vi "Go to Localize.vi"(8 "error in (no error)":errorcluster, 11 "CommonState in":refnum<class "CoordinatorState.lvclass">) -> (0 "error out":errorcluster, 3 "CommonState out":refnum<class "State Actor.lvclass">)   [LabVIEW 2014, in "States.lvlib" / "CoordinatorState.lvclass"]
uses:
  CoordinatorState.lvclass
  <vilib>/NI/Actors/State Actor/State Actor/State Actor.lvclass
  Localize/Localize.lvclass
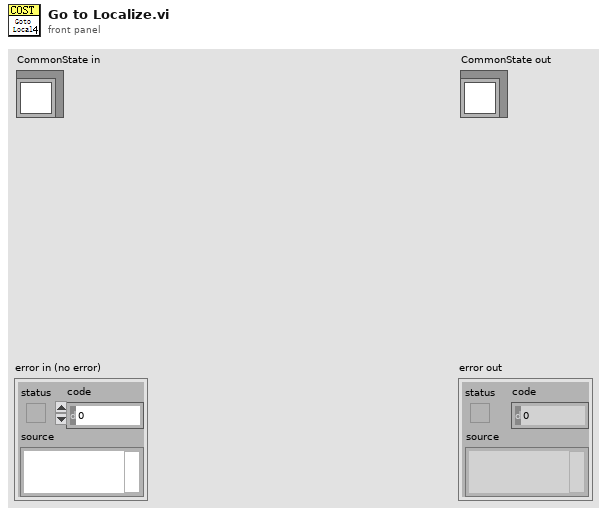
[diagram p1: front panel]
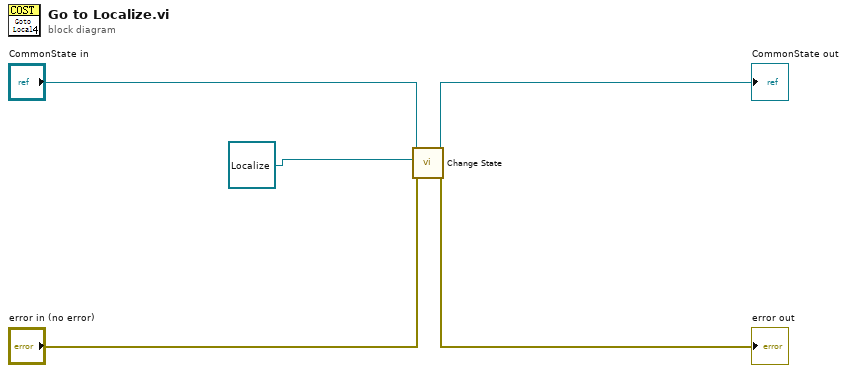
[diagram p0: block diagram]
diagram:
  n1 = call <vilib>:"Change State.vi"("error in (no error)"="error in (no error)", "New State in"=refnum<class "Localize.lvclass"> refnum ("States.lvlib:Localize.lvclass"), "State in"="CommonState in") -> ("error out"=→"error out":errorcluster, "State out"=→"CommonState out":refnum<class "State Actor.lvclass">)  [unwired: 7 in]
